vi "MainGui.Buttons.Update.vi"(7 "Btns":refnum<vi>[](array[refnum]), 8 "error in (no error)":errorcluster, 10 "Mode":T1) -> (0 "error out":errorcluster)   [LabVIEW 2016]
uses:
  Sequence/Sequence.MainMode.ctl
  MainGui.ButtonType.ctl
  Sequence/Sequence.Test.BreakReason.ctl
  Station/Station.Global.vi
  Global/ApplicationGlobal.vi
  Sequence/Sequence.Global.vi
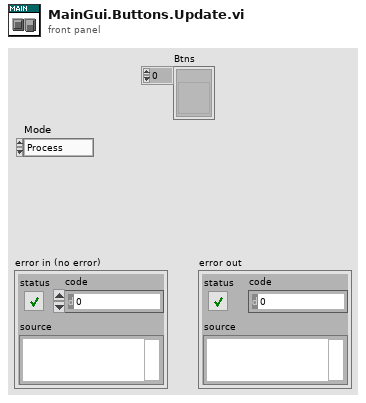
[diagram p1: front panel]
types:
  T1 = typedef "Sequence.MainMode.ctl" = enum16{"Process", "Base", "Order", "Manual", "Logs", "Results", "Stats", "DMC Config"}
  T2 = typedef "Sequence.Data.ctl" = cluster{"BeginTS":timestamp, "EndTS":timestamp, "State":T3, "Status.Work":T4, "Status.Process":T4, "Status.Home":T4, "Status.Wabco":T4, "Status.Client":T4, "BreakReason":T5, "BreakSource":T6, "DoorLock":bool, "Status.Prod":T7[], "UserAction":T11, "UserData":T12, "Error":errorcluster, "Code":T14, "Rotations":i32, "ProdIdx":i32, "ProdDone":T7[], "PrintedSerials-Wabco":i32[], "PrintedSerials-Client":i32[], "Counters-Wabco":T21, "Counters-Client":T21}
  T3 = typedef "Sequence.State.ctl" = enum16{"Init", "Idle", "Home", "Work", "Run", "Pause"}
  T4 = typedef "Sequence.Step.Status.ctl" = enum16{"-", "Pending", "Running", "Skipped", "Passed", "Failed", "Done", "Error", "Aborted", "Stopped"}
  T5 = typedef "Sequence.Test.BreakReason.ctl" = enum16{"-", "NOK container", "OK container", "Rev empty", "Rev missing", "Rev wrong", "Fork missing", "Fork wrong", "NOK limit", "Unload failure", "Single slot", "Part done", "Err: Prod move work", "Err: Prod move home", "Err: Prod lift work", "Err: Prod lift home", "Err: Prod Arm Work", "Err: Prod Arm NOK", "Err: Prod Arm OK", "Err: Prod NOK suck", "Err: Prod NOK drop", "Err: Prod OK missing", "Err: Prod OK suck", "Err: Prod OK drop"}
  T6 = typedef "Sequence.Test.BreakSource.ctl" = enum16{"-", "A", "B", "A/B"}
  T7 = typedef "Sequence.Test.Status.ctl" = cluster{"Slot":T8, "A":T10, "B":T10}
  T8 = typedef "Sequence.Slot.StatusData.ctl" = cluster{"ID":i32, "Unload":T9, "TS":timestamp, "duration":u32}
  T9 = typedef "Sequence.Test.Unload.Status.ctl" = enum16{"init", "check NOK", "check OK", "wait on NOK", "wait on OK", "wait on Unload", "done"}
  T10 = typedef "Sequence.Prod.StatusData.ctl" = cluster{"status":T4, "pause":T5, "present":bool, "printed":bool, "scanned":bool, "tuned":bool, "removed":bool, "OCRignored":bool, "LaserVariables":string[], "Serial":i32, "path":path, "corners":cluster{"X":i32, "Y":i32}[], "verification":u8, "ScanerReadOut":string[]}
  T11 = typedef "Sequence.UserActions.ctl" = cluster{"Stop":bool, "Pause":bool, "Next":bool}
  T12 = typedef "Sequence.UserData.ctl" = cluster{"GuiMode":T1, "Test":T13, "ContinueOrder":bool}
  T13 = typedef "MainGui.TestOptions.ctl" = cluster{"IgnoreResults":bool, "IgnoreImages":bool, "ServiceMode":bool}
  T14 = typedef "Sequence.Code.Sets.ctl" = cluster{"Ready":bool, "DoubleOrder":bool, "OrderDone":bool, "AllowSingleSlot":bool, "IgnoreOCR":bool, "ThresholdA":u8, "ThresholdB":u8, "Plate":T15, "ImgPath":path, "Variant":T16}
  T15 = typedef "Sequence.PlateType.ctl" = enum16{"Wabco", "Client"}
  T16 = typedef "Logger.Variant.Sets.ctl" = cluster{"State":T17, "ImgPath":path, "WabcoPlate":string, "WabcoProduct":string, "ClientProduct":string, "ClientPlate":string, "TotalQuantity":u16, "OrderQuantity":u16, "Serial":i32, "Wabco":T18, "Client":T18}
  T17 = typedef "Station.Changeover.State.vi" = enum16{"Init", "Scaning", "NOK", "Wait for ack", "Ready"}
  T18 = typedef "Station.Plate.Properties.ctl" = cluster{"LaserJob":string, "AdditionalTxt":string, "FactoryCode":string, "RevID":u8, "ForkID":u8, "FailuresLimit":u16, "GlobalCnt":i32, "ScannerProgram":u8, "SerialFormat":T19, "CoordA":T20, "CoordB":T20, "DMCconfig":i32, "CVX_Program":u16}
  T19 = typedef "Sequence.Code.SerialFormat.ctl" = enum8{"", "6 dig", "7 dig"}
  T20 = typedef "V7310.Job.Sets.ctl" = cluster{"X":dbl, "Y":dbl, "Angle":dbl}
  T21 = typedef "Sequence.Counters.ctl" = cluster{"Expected":u16, "Done":u16, "OK":u16, "NOK":u16, "NOKlimit":u16, "Part":u16, "PartOK":u16}
  T22 = typedef "Station.Data.ctl" = cluster{"State":T23, "Seq.State":T3, "Seq.BreakReason":T5, "Seq.BreakSource":T6, "Hw failure":bool, "Unconfirmed":bool, "Station empty":bool, "Home err":bool, "Order done":bool, "DUT present":T24, "EmgState":T25, "Sets":T12, "StatusBits":T26}
  T23 = typedef "Station.State.ctl" = enum16{"Idle", "Ready", "Run", "Stop", "Error", "Home", "Done", "Emg"}
  T24 = typedef "FestoCPX.Station.ProdPresent.ctl" = cluster{"Slot1":cluster{"A":bool, "B":bool}, "Slot2":cluster{"A":bool, "B":bool}, "Slot3":cluster{"A":bool, "B":bool}, "Slot4":cluster{"A":bool, "B":bool}, "Final":cluster{"A":bool, "B":bool}, "OK":cluster{"A":bool, "B":bool}, "Container":cluster{"OK":bool, "NOK":bool}}
  T25 = typedef "FestoCPX.Station.EmgState.ctl" = cluster{"Button":bool, "SideDoor":bool, "FrontDoor":bool, "DoorSecured":bool}
  T26 = typedef "Station.Home.Status.Bits.ctl" = cluster{"Door Close":bool, "Rev OK":bool, "Fork OK":bool, "Container OK":bool, "Station empty":bool}
  T27 = typedef "MainGui.ButtonType.ctl" = enum32{"Exit", "Mode", "Process", "Base", "Order", "Manual", "Logs", "Results", "Accept", "Reject", "Start", "Stop", "Next", "Pause", "Lock", "ManualView", "DoorLock", "Scan", "Select", "ScannerGui", "Stats"}
  T28 = enum8{"Enabled", "Disabled", "Disabled and Grayed Out"}
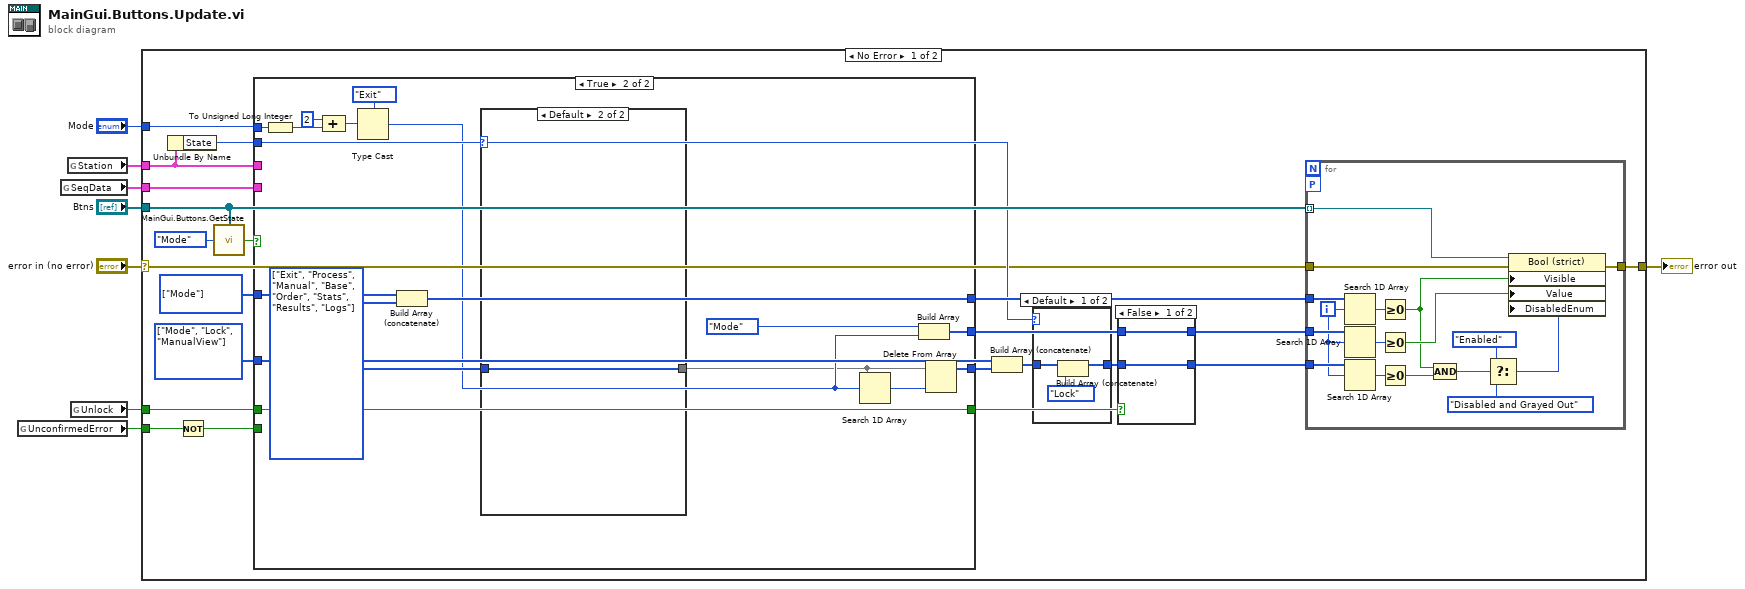
[diagram p0: block diagram]
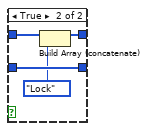
[diagram p3: hidden frame]
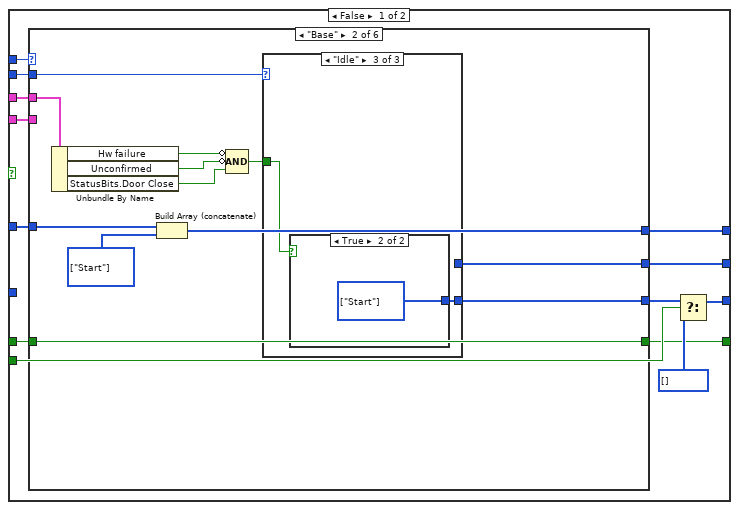
[diagram p4: hidden frame]
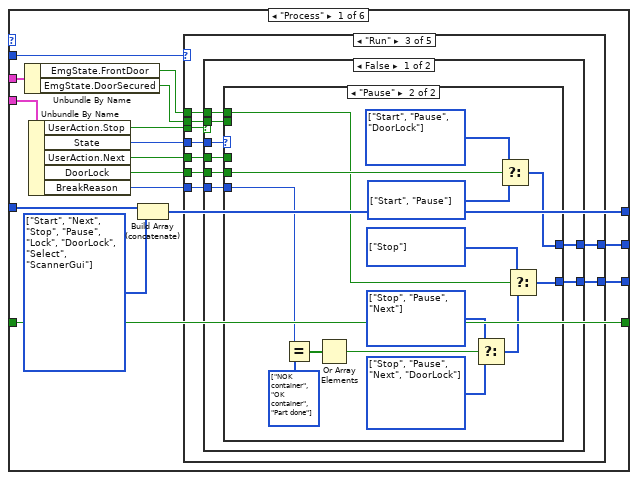
[diagram p5: hidden frame]
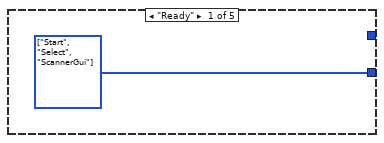
[diagram p6: hidden frame]
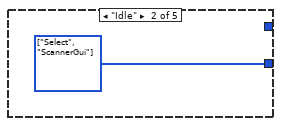
[diagram p7: hidden frame]
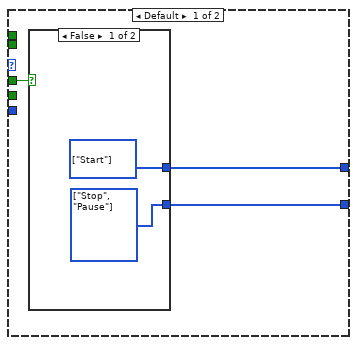
[diagram p8: hidden frame]
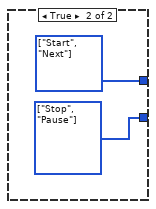
[diagram p9: hidden frame]
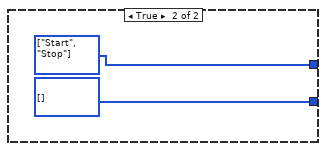
[diagram p10: hidden frame]
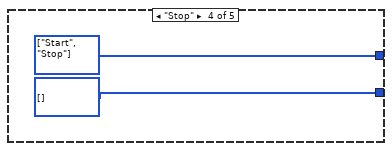
[diagram p11: hidden frame]
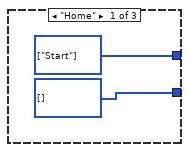
[diagram p13: hidden frame]
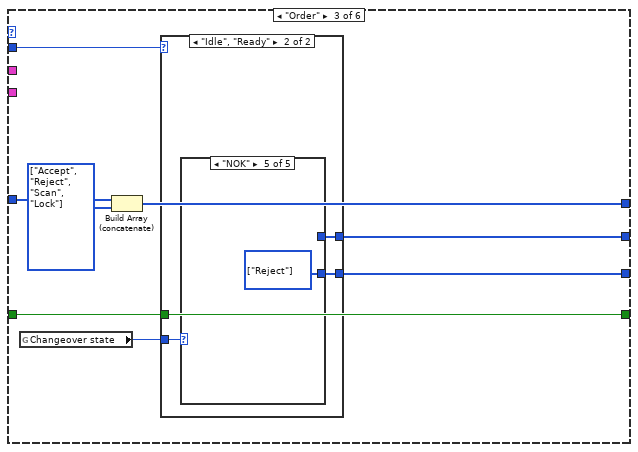
[diagram p16: hidden frame]
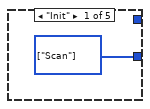
[diagram p18: hidden frame]
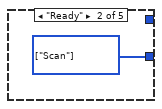
[diagram p19: hidden frame]
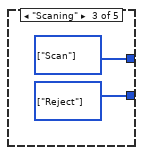
[diagram p20: hidden frame]
diagram:
  n1 = global read "ApplicationGlobal.vi" "UnconfirmedError"() -> (w3:bool)
  n2 = global read "Sequence.Global.vi" "SeqData"() -> (w2:T2)
  n3 = global read "Station.Global.vi" "Station"() -> (w4:T22)
  n4 = global read "ApplicationGlobal.vi" "Unlock"() -> (w1:bool)
  n5 = case shown="No Error" "error in (no error)" {
    selector: "error in (no error)" -> [w16 w205]
    tunnel: "Mode" -> [w30 _]
    tunnel: [w15 w205] -> w7
    tunnel: "Btns" -> [w26 _]
    tunnel: w4 -> [w19 _]
    tunnel: w3 -> [w22 _]
    tunnel: w2 -> [w11 _]
    tunnel: w1 -> [w9 _]
    frame No Error {
      w24 = T27[] [enum."Mode", enum."Lock", enum."ManualView"] items=["Exit", "Mode", "Process", "Base", "Order", "Manual", "Logs", "Results", "Accept", "Reject", "Start", "Stop", "Next", "Pause", "Lock", "ManualView", "DoorLock", "Scan", "Select", "ScannerGui", "Stats"]
      w25 = T27[] [enum."Mode"] items=["Exit", "Mode", "Process", "Base", "Order", "Manual", "Logs", "Results", "Accept", "Reject", "Start", "Stop", "Next", "Pause", "Lock", "ManualView", "DoorLock", "Scan", "Select", "ScannerGui", "Stats"]
      n6 = Unbundle By Name(w19) -> ("State"=w17:T23)
      n7 = Not(x=w22) -> (.not. x?=w21:bool)
      n8 = call "MainGui.Buttons.GetState.vi"("Button"=MainGui.ButtonType."Mode", "Btns"=w26) -> ("State"=w27:bool)
      n9 = case shown="True" w27 {
        tunnel: w30 -> [w70 w200]
        tunnel: [w69 w197] -> w29
        tunnel: w25 -> [w68 w198]
        tunnel: [w67 w187] -> w20
        tunnel: [w63 w192] -> w23
        tunnel: w24 -> [_ _]
        tunnel: w19 -> [w66 _]
        tunnel: w21 -> [w64 _]
        tunnel: w9 -> [w61 w185]
        tunnel: w17 -> [w60 w186]
        tunnel: w11 -> [w59 _]
        tunnel: [w58 w185] -> w10
        frame False {
          w62 = T27[] [] items=["Exit", "Mode", "Process", "Base", "Order", "Manual", "Logs", "Results", "Accept", "Reject", "Start", "Stop", "Next", "Pause", "Lock", "ManualView", "DoorLock", "Scan", "Select", "ScannerGui", "Stats"] ("f")
          n10 = case shown="\"Base\"" w70 {
            tunnel: [w86 w141 w154 w171 w175 w183] -> w69
            tunnel: w68 -> [w85 w142 w155 w172 w176 w184]
            tunnel: [w84 w139 w149 _ _ w179] -> w67
            tunnel: [w83 w138 w152 w166 w173 _] -> w65
            tunnel: w66 -> [w76 w137 _ _ _ _]
            tunnel: w61 -> [w71 w131 w148 _ w174 w177]
            tunnel: w60 -> [w81 w132 w151 _ _ _]
            tunnel: w59 -> [w80 _ _ _ _ _]
            tunnel: [w71 w131 w148 w165 w174 w177] -> w58
            frame "Process" {
              w77 = T27[] [enum."Start", enum."Next", enum."Stop", enum."Pause", enum."Lock", enum."DoorLock", enum."Select", enum."ScannerGui"] items=["Exit", "Mode", "Process", "Base", "Order", "Manual", "Logs", "Results", "Accept", "Reject", "Start", "Stop", "Next", "Pause", "Lock", "ManualView", "DoorLock", "Scan", "Select", "ScannerGui", "Stats"]
              n11 = Unbundle By Name(w76) -> ("EmgState.FrontDoor"=w75:bool, "EmgState.DoorSecured"=w74:bool)
              n12 = Unbundle By Name(w80) -> ("UserAction.Stop"=w82:bool, "State"=w79:T3, "UserAction.Next"=w78:bool, "DoorLock"=w73:bool, "BreakReason"=w72:T5)
              n13 = Build Array (concatenate)(w85, w77) -> (w86:T27[])
              n14 = case shown="\"Run\"" w81 {
                tunnel: [_ _ w97 w130 _] -> w84
                tunnel: [w87 w88 w96 w129 _] -> w83
                tunnel: w82 -> [_ _ w95 _ _]
                tunnel: w79 -> [_ _ w94 _ _]
                tunnel: w78 -> [_ _ w93 _ _]
                tunnel: w75 -> [_ _ w92 _ _]
                tunnel: w74 -> [_ _ w91 _ _]
                tunnel: w73 -> [_ _ w90 _ _]
                tunnel: w72 -> [_ _ w89 _ _]
                frame "Ready" {
                  w87 = T27[] [enum."Start", enum."Select", enum."ScannerGui"] items=["Exit", "Mode", "Process", "Base", "Order", "Manual", "Logs", "Results", "Accept", "Reject", "Start", "Stop", "Next", "Pause", "Lock", "ManualView", "DoorLock", "Scan", "Select", "ScannerGui", "Stats"]
                }
                frame "Idle" {
                  w88 = T27[] [enum."Select", enum."ScannerGui"] items=["Exit", "Mode", "Process", "Base", "Order", "Manual", "Logs", "Results", "Accept", "Reject", "Start", "Stop", "Next", "Pause", "Lock", "ManualView", "DoorLock", "Scan", "Select", "ScannerGui", "Stats"]
                }
                frame "Run" {
                  n15 = case shown="False" w95 {
                    tunnel: [w105 w128] -> w97
                    tunnel: [w104 w127] -> w96
                    tunnel: w94 -> [w103 _]
                    tunnel: w93 -> [w102 _]
                    tunnel: w92 -> [w101 _]
                    tunnel: w91 -> [w100 _]
                    tunnel: w90 -> [w99 _]
                    tunnel: w89 -> [w98 _]
                    frame False {
                      n16 = case shown="\"Pause\"" w103 {
                        tunnel: [w108 w123] -> w105
                        tunnel: [w107 w120] -> w104
                        tunnel: w102 -> [w106 _]
                        tunnel: w101 -> [_ w122]
                        tunnel: w100 -> [_ _]
                        tunnel: w99 -> [_ w124]
                        tunnel: w98 -> [_ w119]
                        frame Default {
                          n17 = case shown="False" w106 {
                            tunnel: [w110 w112] -> w108
                            tunnel: [w109 w111] -> w107
                            frame False {
                              w109 = T27[] [enum."Stop", enum."Pause"] items=["Exit", "Mode", "Process", "Base", "Order", "Manual", "Logs", "Results", "Accept", "Reject", "Start", "Stop", "Next", "Pause", "Lock", "ManualView", "DoorLock", "Scan", "Select", "ScannerGui", "Stats"]
                              w110 = T27[] [enum."Start"] items=["Exit", "Mode", "Process", "Base", "Order", "Manual", "Logs", "Results", "Accept", "Reject", "Start", "Stop", "Next", "Pause", "Lock", "ManualView", "DoorLock", "Scan", "Select", "ScannerGui", "Stats"]
                            }
                            frame True {
                              w111 = T27[] [enum."Stop", enum."Pause"] items=["Exit", "Mode", "Process", "Base", "Order", "Manual", "Logs", "Results", "Accept", "Reject", "Start", "Stop", "Next", "Pause", "Lock", "ManualView", "DoorLock", "Scan", "Select", "ScannerGui", "Stats"]
                              w112 = T27[] [enum."Start", enum."Next"] items=["Exit", "Mode", "Process", "Base", "Order", "Manual", "Logs", "Results", "Accept", "Reject", "Start", "Stop", "Next", "Pause", "Lock", "ManualView", "DoorLock", "Scan", "Select", "ScannerGui", "Stats"]
                            }
                          }
                        }
                        frame "Pause" {
                          w118 = T5[] [enum."NOK container", enum."OK container", enum."Part done"] items=["-", "NOK container", "OK container", "Rev empty", "Rev missing", "Rev wrong", "Fork missing", "Fork wrong", "NOK limit", "Unload failure", "Single slot", "Part done", "Err: Prod move work", "Err: Prod move home", "Err: Prod lift work", "Err: Prod lift home", "Err: Prod Arm Work", "Err: Prod Arm NOK", "Err: Prod Arm OK", "Err: Prod NOK suck", "Err: Prod NOK drop", "Err: Prod OK missing", "Err: Prod OK suck", "Err: Prod OK drop"]
                          w115 = T27[] [enum."Stop", enum."Pause", enum."Next"] items=["Exit", "Mode", "Process", "Base", "Order", "Manual", "Logs", "Results", "Accept", "Reject", "Start", "Stop", "Next", "Pause", "Lock", "ManualView", "DoorLock", "Scan", "Select", "ScannerGui", "Stats"]
                          w114 = T27[] [enum."Stop", enum."Pause", enum."Next", enum."DoorLock"] items=["Exit", "Mode", "Process", "Base", "Order", "Manual", "Logs", "Results", "Accept", "Reject", "Start", "Stop", "Next", "Pause", "Lock", "ManualView", "DoorLock", "Scan", "Select", "ScannerGui", "Stats"]
                          w121 = T27[] [enum."Stop"] items=["Exit", "Mode", "Process", "Base", "Order", "Manual", "Logs", "Results", "Accept", "Reject", "Start", "Stop", "Next", "Pause", "Lock", "ManualView", "DoorLock", "Scan", "Select", "ScannerGui", "Stats"]
                          w126 = T27[] [enum."Start", enum."Pause", enum."DoorLock"] items=["Exit", "Mode", "Process", "Base", "Order", "Manual", "Logs", "Results", "Accept", "Reject", "Start", "Stop", "Next", "Pause", "Lock", "ManualView", "DoorLock", "Scan", "Select", "ScannerGui", "Stats"]
                          w125 = T27[] [enum."Start", enum."Pause"] items=["Exit", "Mode", "Process", "Base", "Order", "Manual", "Logs", "Results", "Accept", "Reject", "Start", "Stop", "Next", "Pause", "Lock", "ManualView", "DoorLock", "Scan", "Select", "ScannerGui", "Stats"]
                          n18 = Equal?(x=w119, y=w118) -> (x = y?=w117:bool[])
                          n19 = Or Array Elements(Boolean array=w117) -> (logical OR=w116:bool)
                          n20 = Select(t=w115, s=w116, f=w114) -> (s? t:f=w113:T27[])
                          n21 = Select(t=w126, s=w124, f=w125) -> (s? t:f=w123:T27[])
                          n22 = Select(t=w121, s=w122, f=w113) -> (s? t:f=w120:T27[])
                        }
                      }
                    }
                    frame True {
                      w127 = T27[] [] items=["Exit", "Mode", "Process", "Base", "Order", "Manual", "Logs", "Results", "Accept", "Reject", "Start", "Stop", "Next", "Pause", "Lock", "ManualView", "DoorLock", "Scan", "Select", "ScannerGui", "Stats"]
                      w128 = T27[] [enum."Start", enum."Stop"] items=["Exit", "Mode", "Process", "Base", "Order", "Manual", "Logs", "Results", "Accept", "Reject", "Start", "Stop", "Next", "Pause", "Lock", "ManualView", "DoorLock", "Scan", "Select", "ScannerGui", "Stats"]
                    }
                  }
                }
                frame "Stop" {
                  w129 = T27[] [] items=["Exit", "Mode", "Process", "Base", "Order", "Manual", "Logs", "Results", "Accept", "Reject", "Start", "Stop", "Next", "Pause", "Lock", "ManualView", "DoorLock", "Scan", "Select", "ScannerGui", "Stats"]
                  w130 = T27[] [enum."Start", enum."Stop"] items=["Exit", "Mode", "Process", "Base", "Order", "Manual", "Logs", "Results", "Accept", "Reject", "Start", "Stop", "Next", "Pause", "Lock", "ManualView", "DoorLock", "Scan", "Select", "ScannerGui", "Stats"]
                }
                frame Default {
                }
              }
            }
            frame "Base" {
              w140 = T27[] [enum."Start"] items=["Exit", "Mode", "Process", "Base", "Order", "Manual", "Logs", "Results", "Accept", "Reject", "Start", "Stop", "Next", "Pause", "Lock", "ManualView", "DoorLock", "Scan", "Select", "ScannerGui", "Stats"]
              n23 = Unbundle By Name(w137) -> ("Hw failure"=w135:bool, "Unconfirmed"=w134:bool, "StatusBits.Door Close"=w133:bool)
              n24 = Build Array (concatenate)(w142, w140) -> (w141:T27[])
              n25 = Compound Arithmetic op=AND(invert w135, invert w134, w133) -> (w136:bool)
              n26 = case shown="\"Idle\"" w132 {
                tunnel: [w144 _ _] -> w139
                tunnel: [w143 _ w146] -> w138
                tunnel: w136 -> [_ _ w145]
                frame "Home" {
                  w143 = T27[] [] items=["Exit", "Mode", "Process", "Base", "Order", "Manual", "Logs", "Results", "Accept", "Reject", "Start", "Stop", "Next", "Pause", "Lock", "ManualView", "DoorLock", "Scan", "Select", "ScannerGui", "Stats"]
                  w144 = T27[] [enum."Start"] items=["Exit", "Mode", "Process", "Base", "Order", "Manual", "Logs", "Results", "Accept", "Reject", "Start", "Stop", "Next", "Pause", "Lock", "ManualView", "DoorLock", "Scan", "Select", "ScannerGui", "Stats"]
                }
                frame "Run", "Emg", Default {
                }
                frame "Idle" {
                  n27 = case shown="True" w145 {
                    tunnel: [_ w147] -> w146
                    frame False {
                    }
                    frame True {
                      w147 = T27[] [enum."Start"] items=["Exit", "Mode", "Process", "Base", "Order", "Manual", "Logs", "Results", "Accept", "Reject", "Start", "Stop", "Next", "Pause", "Lock", "ManualView", "DoorLock", "Scan", "Select", "ScannerGui", "Stats"]
                    }
                  }
                }
              }
            }
            frame "Order" {
              w153 = T27[] [enum."Accept", enum."Reject", enum."Scan", enum."Lock"] items=["Exit", "Mode", "Process", "Base", "Order", "Manual", "Logs", "Results", "Accept", "Reject", "Start", "Stop", "Next", "Pause", "Lock", "ManualView", "DoorLock", "Scan", "Select", "ScannerGui", "Stats"]
              n28 = global read "Station.Global.vi" "Changeover state"() -> (w150:T17)
              n29 = Build Array (concatenate)(w155, w153) -> (w154:T27[])
              n30 = case shown="\"Idle\", \"Ready\"" w151 {
                tunnel: [_ w156] -> w152
                tunnel: w148 -> [_ _]
                tunnel: w150 -> [_ w158]
                tunnel: [_ w157] -> w149
                frame Default {
                }
                frame "Idle", "Ready" {
                  n31 = case shown="\"NOK\"" w158 {
                    tunnel: [_ _ w162 _ _] -> w157
                    tunnel: [w159 w160 w161 w163 w164] -> w156
                    frame "Init" {
                      w159 = T27[] [enum."Scan"] items=["Exit", "Mode", "Process", "Base", "Order", "Manual", "Logs", "Results", "Accept", "Reject", "Start", "Stop", "Next", "Pause", "Lock", "ManualView", "DoorLock", "Scan", "Select", "ScannerGui", "Stats"]
                    }
                    frame "Ready" {
                      w160 = T27[] [enum."Scan"] items=["Exit", "Mode", "Process", "Base", "Order", "Manual", "Logs", "Results", "Accept", "Reject", "Start", "Stop", "Next", "Pause", "Lock", "ManualView", "DoorLock", "Scan", "Select", "ScannerGui", "Stats"]
                    }
                    frame "Scaning" {
                      w161 = T27[] [enum."Reject"] items=["Exit", "Mode", "Process", "Base", "Order", "Manual", "Logs", "Results", "Accept", "Reject", "Start", "Stop", "Next", "Pause", "Lock", "ManualView", "DoorLock", "Scan", "Select", "ScannerGui", "Stats"]
                      w162 = T27[] [enum."Scan"] items=["Exit", "Mode", "Process", "Base", "Order", "Manual", "Logs", "Results", "Accept", "Reject", "Start", "Stop", "Next", "Pause", "Lock", "ManualView", "DoorLock", "Scan", "Select", "ScannerGui", "Stats"]
                    }
                    frame "Wait for ack" {
                      w163 = T27[] [enum."Accept", enum."Reject"] items=["Exit", "Mode", "Process", "Base", "Order", "Manual", "Logs", "Results", "Accept", "Reject", "Start", "Stop", "Next", "Pause", "Lock", "ManualView", "DoorLock", "Scan", "Select", "ScannerGui", "Stats"]
                    }
                    frame "NOK" {
                      w164 = T27[] [enum."Reject"] items=["Exit", "Mode", "Process", "Base", "Order", "Manual", "Logs", "Results", "Accept", "Reject", "Start", "Stop", "Next", "Pause", "Lock", "ManualView", "DoorLock", "Scan", "Select", "ScannerGui", "Stats"]
                    }
                  }
                }
              }
            }
            frame "DMC Config" {
              w169 = T27[] [enum."Reject", enum."Lock"] items=["Exit", "Mode", "Process", "Base", "Order", "Manual", "Logs", "Results", "Accept", "Reject", "Start", "Stop", "Next", "Pause", "Lock", "ManualView", "DoorLock", "Scan", "Select", "ScannerGui", "Stats"]
              w168 = T27[] [enum."Accept", enum."Reject", enum."Lock"] items=["Exit", "Mode", "Process", "Base", "Order", "Manual", "Logs", "Results", "Accept", "Reject", "Start", "Stop", "Next", "Pause", "Lock", "ManualView", "DoorLock", "Scan", "Select", "ScannerGui", "Stats"]
              n32 = global read "ApplicationGlobal.vi" "DMCConfig.Unlock"() -> (w165:bool)
              n33 = global read "Station.Global.vi" "DMCchanged2"() -> (w170:bool)
              n34 = Compound Arithmetic op=AND(w170, w165) -> (w167:bool)
              n35 = Select(t=w168, s=w167, f=w169) -> (s? t:f=w166:T27[])
              n36 = Build Array (concatenate)(w172, w168) -> (w171:T27[])
            }
            frame "Logs".."Stats" {
              w173 = T27[] [enum."Results", enum."Logs", enum."Stats"] items=["Exit", "Mode", "Process", "Base", "Order", "Manual", "Logs", "Results", "Accept", "Reject", "Start", "Stop", "Next", "Pause", "Lock", "ManualView", "DoorLock", "Scan", "Select", "ScannerGui", "Stats"]
              n37 = Build Array (concatenate)(w176, w173) -> (w175:T27[])
            }
            frame "Manual" {
              w180 = T27[] [] items=["Exit", "Mode", "Process", "Base", "Order", "Manual", "Logs", "Results", "Accept", "Reject", "Start", "Stop", "Next", "Pause", "Lock", "ManualView", "DoorLock", "Scan", "Select", "ScannerGui", "Stats"] ("f")
              w181 = T27[] [enum."ManualView"] items=["Exit", "Mode", "Process", "Base", "Order", "Manual", "Logs", "Results", "Accept", "Reject", "Start", "Stop", "Next", "Pause", "Lock", "ManualView", "DoorLock", "Scan", "Select", "ScannerGui", "Stats"] ("f")
              w182 = T27[] [enum."Lock", enum."ManualView"] items=["Exit", "Mode", "Process", "Base", "Order", "Manual", "Logs", "Results", "Accept", "Reject", "Start", "Stop", "Next", "Pause", "Lock", "ManualView", "DoorLock", "Scan", "Select", "ScannerGui", "Stats"]
              n38 = Build Array (concatenate)(w184, w182) -> (w183:T27[])
              n39 = global read "ApplicationGlobal.vi" "ManualView"() -> (w178:bool)
              n40 = Select(t=w181, s=w178, f=w180) -> (s? t:f=w179:T27[])
            }
          }
          n41 = Select(t=w65, s=w64, f=w62) -> (s? t:f=w63:T27[])
        }
        frame True {
          w193 = T27[] [enum."Exit", enum."Process", enum."Manual", enum."Base", enum."Order", enum."Stats", enum."Results", enum."Logs"] items=["Exit", "Mode", "Process", "Base", "Order", "Manual", "Logs", "Results", "Accept", "Reject", "Start", "Stop", "Next", "Pause", "Lock", "ManualView", "DoorLock", "Scan", "Select", "ScannerGui", "Stats"]
          n42 = To Unsigned Long Integer(number=w200) -> (unsigned 32bit integer=w199:u32)
          n43 = Compound Arithmetic op=ADD(u32 2 ("value"), w199) -> (w195:u32)
          n44 = Type Cast(type=MainGui.ButtonType."Exit" ("Button"), x=w195) -> (*(type *) &x=w189:T27)
          n45 = Build Array (concatenate)(w198, w193) -> (w197:T27[])
          n46 = case shown="Default" w186 {
            tunnel: w193 -> [w203 w204]
            tunnel: [w201 w204] -> w188
            frame "Run", "Home" {
              n47 = Array Subset(array=w203, index=1) -> (w201:T27[])  [unwired: 1 in]
            }
            frame Default {
            }
          }
          n48 = Search 1D Array(1D array=w188, element=w189) -> (index of element=w191:i32)  [unwired: 1 in]
          n49 = Build Array(MainGui.ButtonType."Mode" ("Button"), w189) -> (w187:T27[])
          n50 = Delete From Array(array=w188, index=w191) -> (array with subset deleted=w192:T27[])  [unwired: 1 in, 1 out]
        }
      }
      n51 = Build Array (concatenate)(w24, w23) -> (w18:T27[])
      n52 = case shown="Default" w17 {
        tunnel: w18 -> [w33 w34]
        tunnel: [w32 w34] -> w14
        frame Default {
          n53 = Build Array (concatenate)(w33, MainGui.ButtonType."Lock" ("Button")) -> (w32:T27[])
        }
        frame "Run" {
        }
      }
      n54 = case shown="False" w10 {
        tunnel: w20 -> [w36 w40]
        tunnel: [w36 w39] -> w12
        tunnel: w14 -> [w35 w38]
        tunnel: [w35 w38] -> w13
        frame False {
        }
        frame True {
          n55 = Build Array (concatenate)(w40, MainGui.ButtonType."Lock" ("Button")) -> (w39:T27[])
        }
      }
      n56 = for {
        tunnel: w26 -> [w57] mode=indexing
        tunnel: w29 -> [w52]
        tunnel: w12 -> [w49]
        tunnel: w13 -> [w46]
        workers-P: _ -> [_]
        tunnel: w16 -> [w42]
        tunnel: [w41] -> w15
        i -> [w43]
        n57 = Search 1D Array(1D array=w52, element=w43) -> (index of element=w51:i32)  [unwired: 1 in]
        n58 = Search 1D Array(1D array=w49, element=w43) -> (index of element=w50:i32)  [unwired: 1 in]
        n59 = Search 1D Array(1D array=w46, element=w43) -> (index of element=w45:i32)  [unwired: 1 in]
        n60 = Greater Or Equal To 0?(x=w51) -> (x >= 0?=w47:bool)
        n61 = Greater Or Equal To 0?(x=w50) -> (x >= 0?=w48:bool)
        n62 = Greater Or Equal To 0?(x=w45) -> (x >= 0?=w44:bool)
        n63 = Compound Arithmetic op=AND(w47, w44) -> (w55:bool)
        n64 = Select(t=T28."Enabled" ("Disabled"), s=w55, f=T28."Disabled and Grayed Out" ("Disabled")) -> (s? t:f=w53:T28)
        n65 = property class="Bool (strict)"(reference=w57, error in=w42, "Visible"=w47, "Value"=w48, "DisabledEnum"=w53) -> (error out=w41:errorcluster)  [unwired: 1 out]
      }
    }
    frame Error {
    }
  }
  "error out" <- w7
